vi "PS3 Controller Test.vi"() -> ()   [LabVIEW 2014]
panel:
  in  "stop":bool
  in  "device ID":i32=3
  out "Arrows":i32
  out "Control cluster":T1 {"Roll" scale=-1.0..1.0; "Pitch" scale=-1.0..1.0; "Vertical Speed" scale=-1.0..1.0; "Yaw Speed" scale=-1.0..1.0}
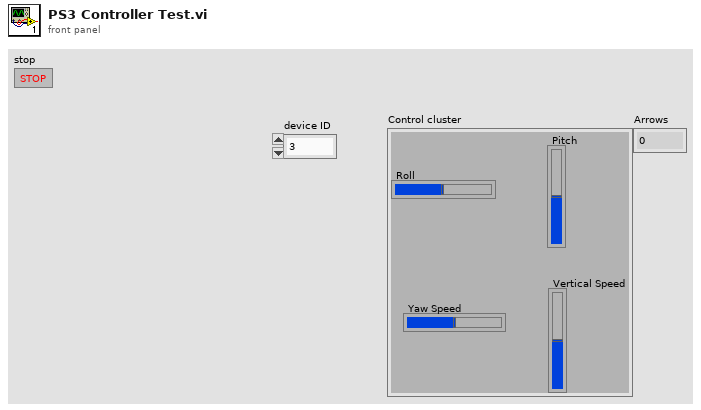
[diagram p1: front panel]
types:
  T1 = cluster{"Roll":dbl, "Pitch":dbl, "Vertical Speed":dbl, "Yaw Speed":dbl}
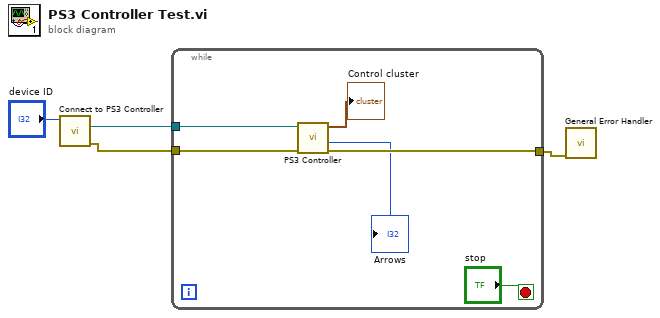
[diagram p0: block diagram]
diagram:
  n1 = call "Connect to PS3 Controller.vi"("device ID"="device ID") -> ("error out"=w3:errorcluster, "device ID 2"=w4:refnum<k1>)  [unwired: 7 in, 1 out]
  n2 = while {
    tunnel: w4 -> [w10]
    tunnel: w3 -> [w9]
    tunnel: [w8] -> w2
    stop <- "stop" stop-if-true
    n3 = call "PS3 Controller.vi"("error in (no error)"=w9, "device ID"=w10) -> ("error out"=w8:errorcluster, "Arrows"=→"Arrows":i32, "Control cluster"=→"Control cluster":T1)  [unwired: 6 in, 1 out]
  }
  n4 = call <vilib>:"General Error Handler.vi"("error in (no error)"=w2) -> ()  [unwired: 10 in, 5 out]
